vi "get chart data.vi"(8 "error in (no error)":errorcluster, 10 "chart_data":T1, 11 "id":i32) -> (0 "error out":errorcluster, 2 "chart_data out":T1, 3 "function return":i32)   [LabVIEW 2012, in "libximc.lvlib"]
doc: "result_t XIMC_API get_chart_data (device_t id, chart_data_t* chart_data);"
uses:
  libximc.lvlib
  libximc.dll
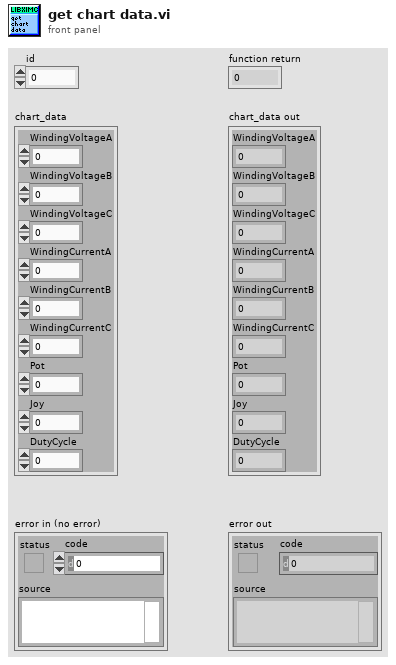
[diagram p1: front panel]
types:
  T1 = cluster{"WindingVoltageA":i32, "WindingVoltageB":i32, "WindingVoltageC":i32, "WindingCurrentA":i32, "WindingCurrentB":i32, "WindingCurrentC":i32, "Pot":u32, "Joy":u32, "DutyCycle":i32}
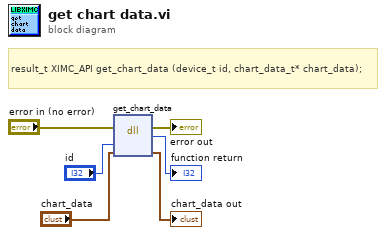
[diagram p0: block diagram]
diagram:
  # "result_t XIMC_API get_chart_data (device_t id, chart_data_t* chart_data);"
  n1 = dll-call lib="E:/labview-2.12.1-Labview_12.0/ximcLVx32/libximc.*" fn="get_chart_data"(error in="error in (no error)", "id"="id", "chart_data"="chart_data") -> (error out=→"error out":errorcluster, →"function return":i32, "chart_data"=→"chart_data out":T1)  [unwired: 3 in, 1 out]
